vi "MJGPID.vi"(8 "PID Gains":cluster{"Kp":dbl, "Kd":dbl, "Ki":dbl}, 10 "Encoder Position":i32, 11 "Reference":dbl) -> (2 "Direction":bool, 3 "Duty Cycle":dbl)   [LabVIEW 2016]
uses:
  IRISSoft LV2016/Library/KevinLibraryAll/labview2011/kevLib2011/Utilities/kCoerceFloat.vi
  IRISSoft LV2016/Library/KevinLibraryAll/labview2011/kevLib2011.lvlib
panel:
  out "Control Input":dbl
  in  "Reverse Motor?":bool
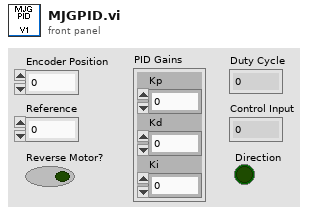
[diagram p1: front panel]
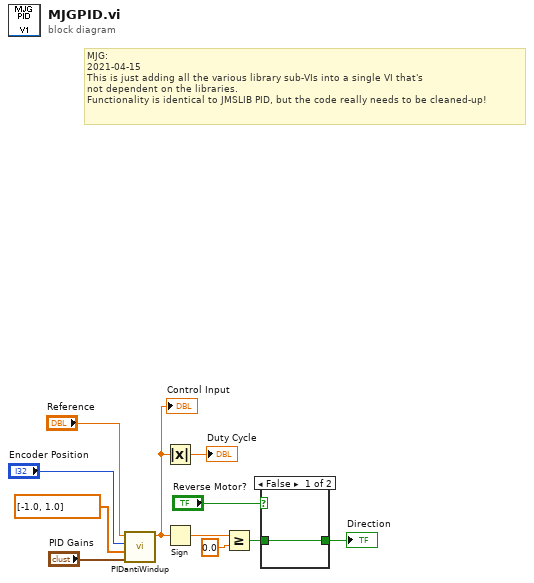
[diagram p0: block diagram]
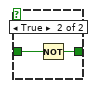
[diagram p2: hidden frame]
diagram:
  # "MJG: \n2021-04-15\nThis is just adding all the various library sub-VIs into a single VI that's \nnot dependent on the libraries. \nFunctionality is identical to JMSLIB PID, but the code really needs to be cleaned-up!"
  n1 = call "PIDantiWindup.vi"("PID Gains"="PID Gains", "Saturation"=dbl[] [-1.0, 1.0], "Position"="Encoder Position", "Reference"="Reference") -> ("control"=w10:dbl)  [unwired: 7 in]
  "Control Input" <- w10
  n2 = Absolute Value(x=w10) -> (abs(x)=→"Duty Cycle":dbl)
  n3 = Sign(1:w10) -> (0:w8:dbl)
  n4 = Greater Or Equal?(x=w8, y=0.0) -> (x >= y?=w2:bool)
  n5 = case shown="False" "Reverse Motor?" {
    tunnel: w2 -> [w12 w14]
    tunnel: [w12 w13] -> w1
    frame False {
    }
    frame True {
      n6 = Not(x=w14) -> (.not. x?=w13:bool)
    }
  }
  "Direction" <- w1
